vi "POST_Multipart_req_PS.vi"(7 "Headers":string, 8 "error in":errorcluster, 9 "Multpart/Form-Data":T1(array[cluster]), 11 "URL":string) -> (0 "error out":errorcluster, 3 "Multipart PATCH Request":string)   [LabVIEW 2016]
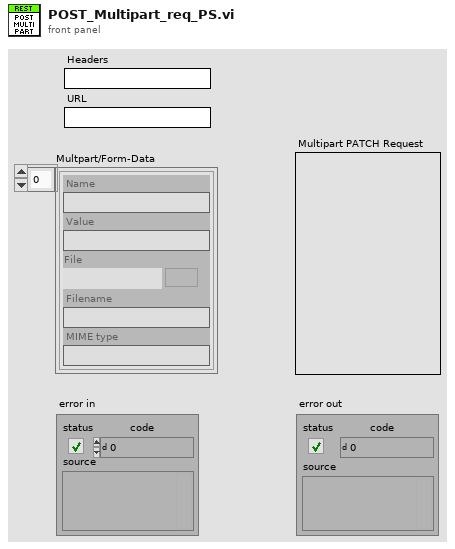
[diagram p1: front panel]
types:
  T1 = cluster{"Name":string, "Value":string, "File":path, "Filename":string, "MIME type":string}[]
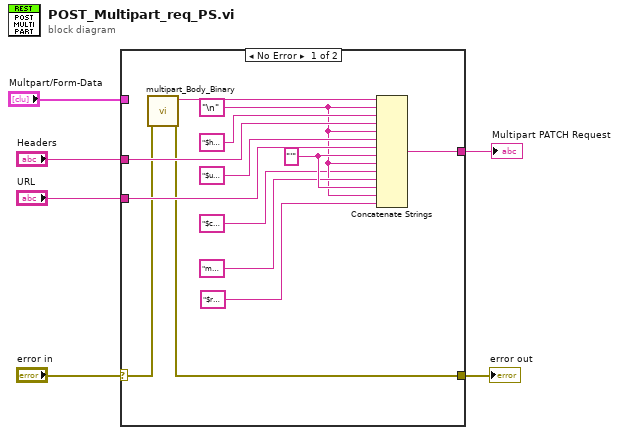
[diagram p0: block diagram]
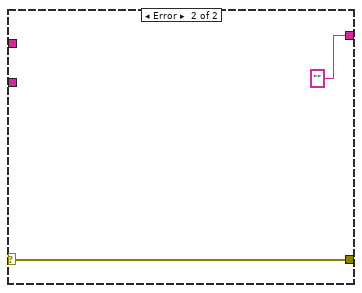
[diagram p2: hidden frame]
diagram:
  n1 = case shown="No Error" "error in" {
    selector: "error in" -> [w8 w20]
    tunnel: "Headers" -> [w19 _]
    tunnel: "URL" -> [w16 _]
    tunnel: [w15 ""] -> w4
    tunnel: [w7 w20] -> w2
    tunnel: "Multpart/Form-Data" -> [_ _]
    frame No Error {
      w14 = "'" ("string")
      w10 = "\n"
      n2 = call "multipart_Body_Binary.vi"("error in"=w8) -> ("error out"=w7:errorcluster, "Multipart Binary Body"=w12:string)  [unwired: 9 in]
      n3 = Concatenate Strings(w12, w10, "$headers = ", w19, w10, "$url = '" ("string"), w16, w14, w10, "$contenttype = '" ("string"), "multipart/form-data; boundary=BlockBoundary", w14, w10, "$request = Invoke-WebRequest -Method 'POST' -Uri $url -Headers $headers -ContentType $contenttype -InFile 'RequestBodySavedToFile' \nRemove-Item RequestBodySavedToFile" ("string")) -> (w15:string)
    }
    frame Error {
    }
  }
  "Multipart PATCH Request" <- w4
  "error out" <- w2
